vi "Skip white spaces.vi"(11 "String":string) -> (2 "1st non-white space":i32, 3 "After white spaces":string)   [LabVIEW 2019]
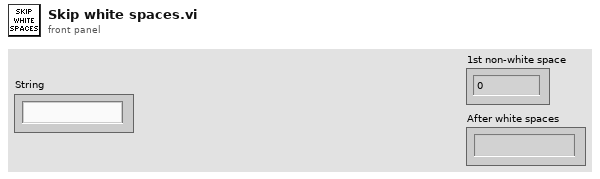
[diagram p1: front panel]
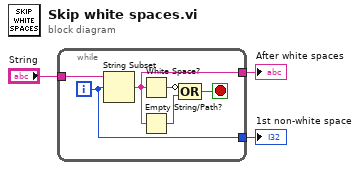
[diagram p0: block diagram]
diagram:
  n1 = while {
    tunnel: "String" -> [w6]
    tunnel: [w5] -> w1
    tunnel: [w4] -> w2
    i -> [w4]
    stop <- w7 stop-if-true
    n2 = String Subset(string=w6, offset (0)=w4) -> (substring=w5:string)  [unwired: 1 in]
    n3 = White Space?(1:w5) -> (0:w9:bool)
    n4 = Empty String/Path?(string/path=w5) -> (empty?=w8:bool)
    n5 = Compound Arithmetic op=OR(invert w9, w8) -> (w7:bool)
  }
  "1st non-white space" <- w2
  "After white spaces" <- w1
